vi "PosNeg.vi"(9 "String":string, 10 "A":dbl, 11 "String 2":string) -> ()   [LabVIEW 2021]
panel:
  out "String 3":string
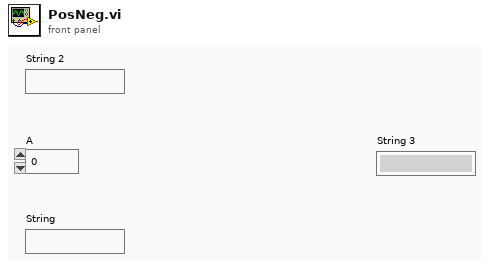
[diagram p1: front panel]
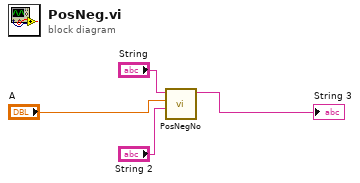
[diagram p0: block diagram]
diagram:
  n1 = call "PosNegNo.vi"("String 2"="String 2", "A"="A", "String"="String") -> ("String 3"=→"String 3":string)  [unwired: 8 in]
